vi "UDP Server Subnet A.vi"(8 "error in (no error)":errorcluster, 9 "Subnet":string, 10 "User Event in":refnum<class "User Event.lvclass">, 11 "UDP Port":u16=5005) -> (0 "error out":errorcluster)   [LabVIEW 2016]
uses:
  User Events/User Event.lvclass
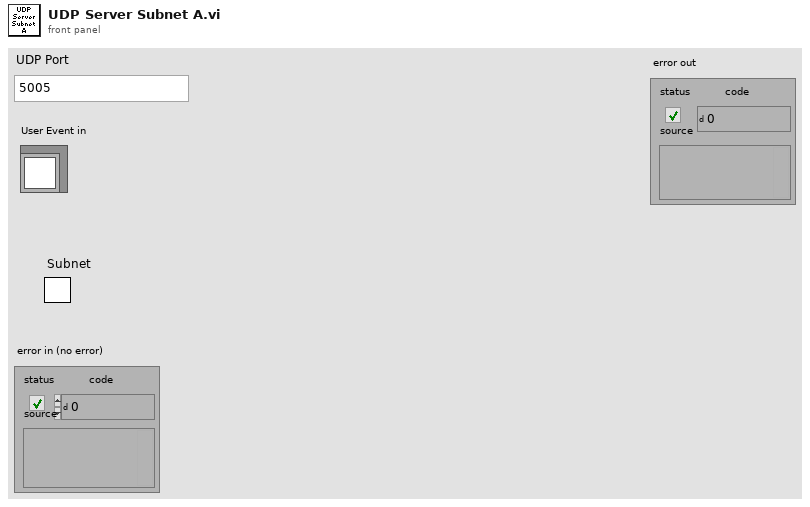
[diagram p1: front panel]
types:
  T1 = typedef "M1M3SupSimUserEvents.ctl" = cluster{"ILCResponse":refnum<user-event>, "StopUDPServer":refnum<user-event>, "InclinometerResponse":refnum<user-event>, "DisplaceResponse":refnum<user-event>, "AccelerometerResponse":refnum<user-event>, "DigitalInput":refnum<user-event>}
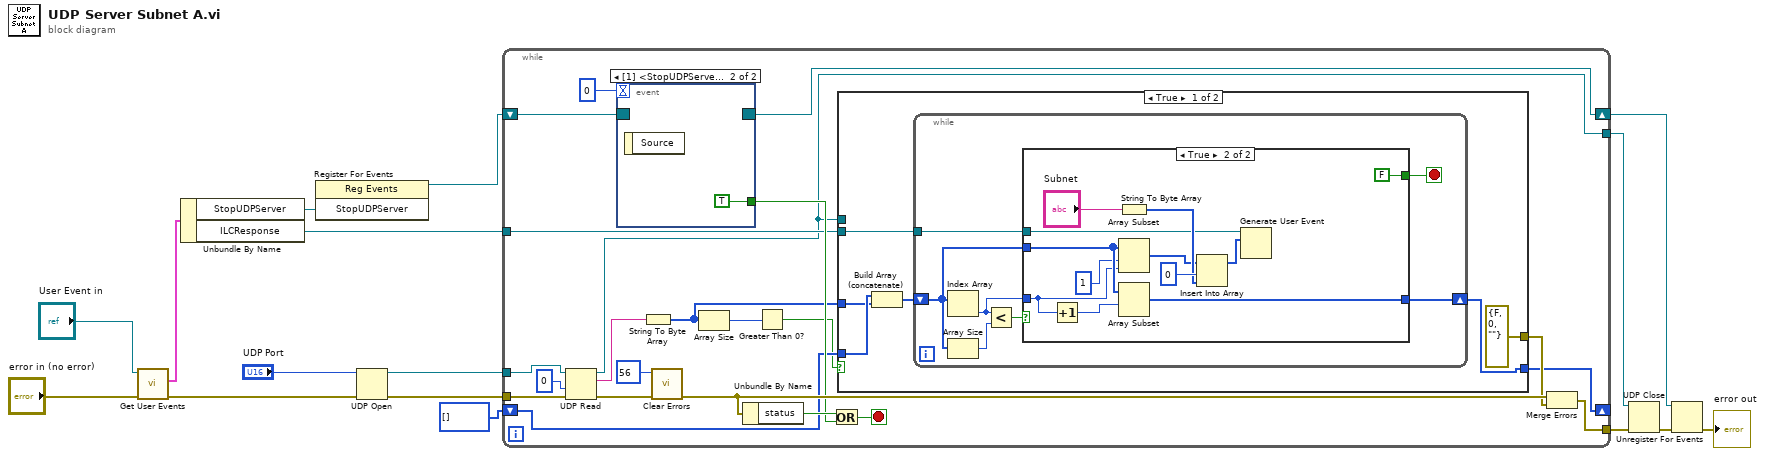
[diagram p0: block diagram]
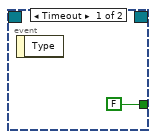
[diagram p2: hidden frame]
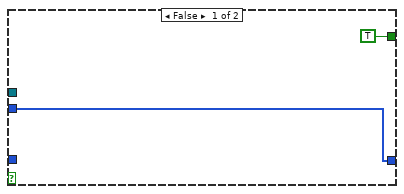
[diagram p3: hidden frame]
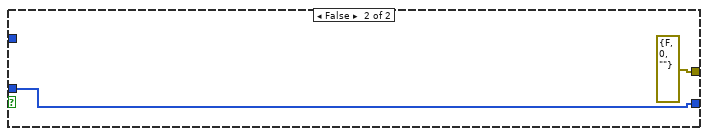
[diagram p4: hidden frame]
diagram:
  n1 = call "Get User Events.vi"("error in (no error)"="error in (no error)", "User Event in"="User Event in") -> ("error out"=w15:errorcluster, "User Events"=w12:T1)  [unwired: 7 in, 1 out]
  n2 = Unbundle By Name(w12) -> ("StopUDPServer"=w13:refnum<user-event>, "ILCResponse"=w16:refnum<user-event>)
  n3 = register-events(w13) -> (reference out=w7:refnum<event-registration>)  [unwired: 2 in, 1 out]
  n4 = UDP Open(8:w15, 11:"UDP Port") -> (port=w3:refnum<k16>, 0:w4:errorcluster)  [unwired: 3 in, 1 out]
  n5 = while {
    tunnel: w3 -> [w38]
    tunnel: w4 -> [w37]
    tunnel: [w30] -> w6
    tunnel: [w23] -> w5
    shift-right: [w25] -> w9
    shift-left: w7 -> [w28]
    tunnel: w16 -> [w24]
    shift-right: [w20] -> _
    shift-left: u8[] [] ("unsigned byte array") -> [w21]
    stop <- w29 stop-if-true
    n6 = UDP Read(connection ID=w38, timeout ms (25000)=0, 8:w37) -> (data out=w22:string, error out=w35:errorcluster, 3:w23:refnum<k16>)  [unwired: 1 in, 2 out]
    n7 = event shown="[1] <StopUDPServer>: User Event" {
      selector: w28 -> [_ _]
      dyn-events: [_ _] -> w25
      timeout: 0 -> [_ _]
      tunnel: [FALSE TRUE] -> w26
      event Timeout {
        n8 = event-data() -> ()  [unwired: 1 in, 1 out]
      }
      event User Event {
        n9 = event-data() -> ()  [unwired: 1 in, 1 out]
      }
    }
    n10 = String To Byte Array(string=w22) -> (unsigned byte array=w19:u8[])
    n11 = call <vilib>:"Clear Errors.vi"("error in (no error)"=w35, "specific error code to clear (0: all)"=56) -> ("error out"=w32:errorcluster)  [unwired: 4 in, 1 out]
    n12 = Array Size(array=w19) -> (size(s)=w18:i32)
    n13 = Unbundle By Name(w32) -> ("status"=w33:bool)
    n14 = Greater Than 0?(x=w18) -> (x > 0?=w17:bool)
    n15 = Or(x=w33, y=w26) -> (x .or. y?=w29:bool)
    n16 = case shown="True" w17 {
      tunnel: [errorcluster {"status"=FALSE, "code"=0, "source"=""} ("error out") errorcluster {"status"=FALSE, "code"=0, "source"=""} ("error out")] -> w31
      tunnel: w24 -> [w43 _]
      tunnel: w23 -> [_ _]
      tunnel: w19 -> [w45 _]
      tunnel: w21 -> [w46 w68]
      tunnel: [w41 w68] -> w20
      frame True {
        n17 = Build Array (concatenate)(w46, w45) -> (w44:u8[])
        n18 = while {
          tunnel: w43 -> [w52]
          shift-right: [w50] -> w41
          shift-left: w44 -> [w49]
          stop <- w51 stop-if-true
          n19 = Index Array(array=w49) -> (element=w47:u8)  [unwired: 1 in]
          n20 = Array Size(array=w49) -> (size(s)=w48:i32)
          n21 = Less?(x=w47, y=w48) -> (x < y?=w53:bool)
          n22 = case shown="True" w53 {
            tunnel: w49 -> [w55 w62]
            tunnel: w47 -> [_ w56]
            tunnel: w52 -> [_ w63]
            tunnel: [w55 w61] -> w50
            tunnel: [TRUE FALSE] -> w51
            frame False {
            }
            frame True {
              n23 = Increment(x=w56) -> (x+1=w57:u8)
              n24 = String To Byte Array(string="Subnet") -> (unsigned byte array=w66:u8[])
              n25 = Array Subset(array=w62, index=1, length=w56) -> (w64:u8[])
              n26 = Array Subset(array=w62, index=w57) -> (w61:u8[])  [unwired: 1 in]
              n27 = Insert Into Array(array=w64, index=0, new element=w66) -> (w59:u8[])
              n28 = Generate User Event(user event=w63, event data cluster=w59) -> ()  [unwired: 2 in, 2 out]
            }
          }
        }
      }
      frame False {
      }
    }
    n29 = Merge Errors(w32, w31) -> (w30:errorcluster)
  }
  n30 = UDP Close(connection ID=w5, 8:w6) -> (error out=w8:errorcluster)  [unwired: 1 out]
  n31 = Unregister For Events(event registration refnum=w9, error in=w8) -> (error out=→"error out":errorcluster)
